vi "ATF-DI Display Filtyer.vi"(10 "DI Data":digitalwaveform[](array[waveform])) -> (2 "DI out":bool[](array[boolean]))   [LabVIEW 2022 SP3]
uses:
  <vilib>/Analysis/3filter.llb/Filter Passband Type.ctl
  <vilib>/Analysis/NI_AALBase.lvlib
  <vilib>/ptbypt/NI_PtbyPt.lvlib
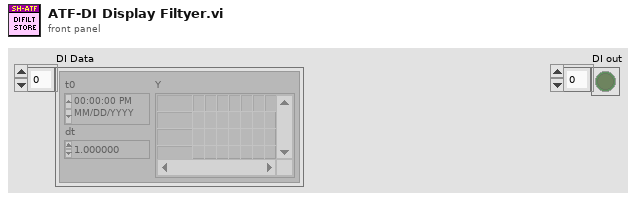
[diagram p1: front panel]
types:
  T1 = typedef "NI_AALBase.lvlib/Filter Passband Type.ctl" = enum32{"Lowpass", "Highpass", "Bandpass", "Bandstop"}
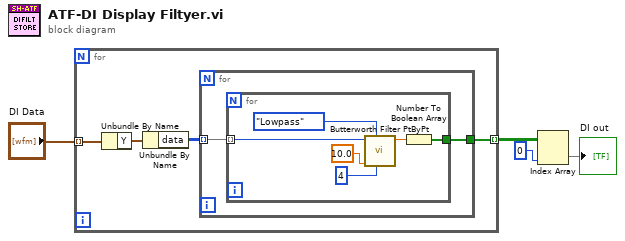
[diagram p0: block diagram]
diagram:
  n1 = for {
    tunnel: "DI Data" -> [w8] mode=indexing
    tunnel: [w5] -> w3 mode=indexing
    n2 = Unbundle By Name(w8) -> ("Y"=w7:digitaldata)
    n3 = Unbundle By Name(w7) -> ("data"=w6:u8[][])
    n4 = for {
      tunnel: w6 -> [w10] mode=indexing
      tunnel: [w9] -> w5
      n5 = for {
        tunnel: w10 -> [w16] mode=indexing
        tunnel: [w11] -> w9
        n6 = call <vilib>:"Butterworth Filter PtByPt.vi"("order"=4, "filter type"=Filter_Passband_Type."Lowpass", "low cutoff freq: fl"=10.0, "x"=w16) -> ("Filtered x"=w12:dbl)  [unwired: 5 in, 1 out]
        n7 = Number To Boolean Array(number=w12) -> (Boolean array=w11:bool[])
      }
    }
  }
  n8 = Index Array(array=w3, index (col)=0 ("disabled index (col)")) -> (element=→"DI out":bool[])  [unwired: 1 in]
